vi "From JPEG Stream.vi"(8 "error in (no error)":errorcluster, 11 "Byte Stream":string) -> (0 "error out":errorcluster, 3 "image data":T1)   [LabVIEW 2020, in "LV Tiff.lvlib"]
uses:
  LV Tiff.lvlib
  <vilib>/picture/picture.llb/imagedata.ctl
  <vilib>/Dataflow_G/G-Image/G-Image.lvlib
  <vilib>/Dataflow_G/G-Image/Image IO/Polymorphic VIs/Load Image (Memory).vi
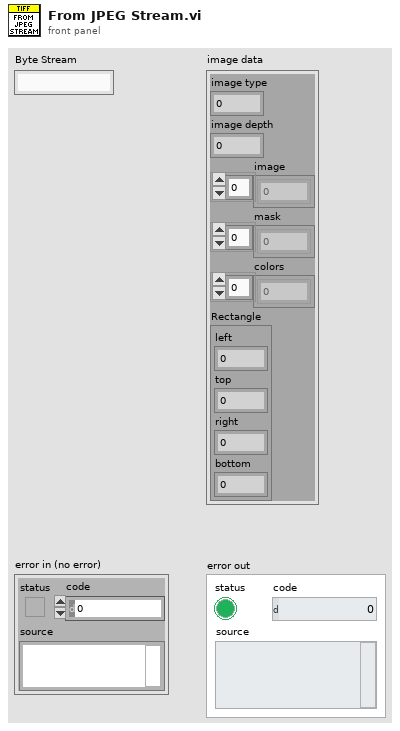
[diagram p1: front panel]
types:
  T1 = typedef "imagedata.ctl" = cluster{"image type":i32, "image depth":i32, "image":u8[], "mask":u8[], "colors":u32[], "Rectangle":cluster{"left":i16, "top":i16, "right":i16, "bottom":i16}}
  T2 = enum16{"open", "replace", "create", "open or create", "replace or create", "replace or create with confirmation"}
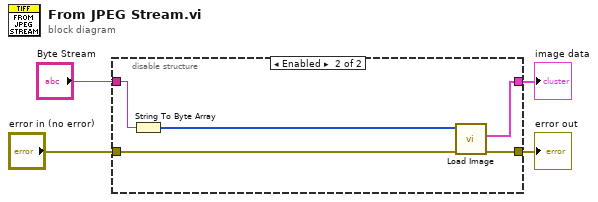
[diagram p0: block diagram]
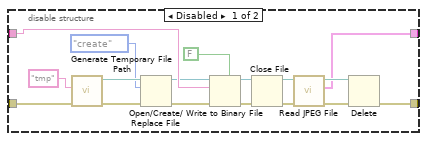
[diagram p2: hidden frame]
diagram:
  n1 = disable-structure shown="Enabled" {
    disable-tunnel: "Byte Stream" -> [w17 w26]
    disable-tunnel: [w7 w22] -> w3
    disable-tunnel: "error in (no error)" -> [w6 w24]
    disable-tunnel: [w5 w23] -> w1
    frame Disabled {
      n2 = call <vilib>:"Generate Temporary File Path.vi"("error in (no error)"=w6, "Temporary File Extension (tmp)"="tmp") -> ("error out"=w19:errorcluster, "Unique Temporary File Path"=w20:path)  [unwired: 8 in]
      n3 = Open/Create/Replace File(file path (use dialog)=w20, error in=w19, operation (0:open)=T2."create") -> (refnum out=w15:refnum<file>, error out=w16:errorcluster)  [unwired: 3 in, 1 out]
      n4 = Write to Binary File(file (use dialog)=w15, data=w17, error in=w16, 5:FALSE ("prepend array or string size? (T)")) -> (refnum out=w13:refnum<file>, error out=w12:errorcluster)  [unwired: 2 in, 1 out]
      n5 = Close File(refnum=w13, error in=w12) -> (path=w11:path, error out=w10:errorcluster)
      n6 = call <vilib>:"Read JPEG File.vi"("error in (no error)"=w10, "path to JPEG file"=w11) -> ("error out"=w9:errorcluster, "image data"=w7:T1, "path"=w8:path)  [unwired: 7 in]
      n7 = Delete(path (use dialog)=w8, error in=w9) -> (error out=w5:errorcluster)  [unwired: 3 in, 2 out]
    }
    frame Enabled {
      n8 = String To Byte Array(string=w26) -> (unsigned byte array=w25:u8[])
      n9 = call-poly <vilib>:"Load Image.vi"("error in (no error)"=w24, "Encoded Image"=w25) -> ("error out"=w23:errorcluster, "Image"=w22:T1)  [unwired: 8 in]
    }
  }
  "image data" <- w3
  "error out" <- w1
